vi "WriteStream ClientStreamTemplate.vi"(8 "error in":errorcluster, 10 "Request Data":cluster{"Numeric":dbl}, 11 "Call ID in":T1) -> (0 "error out":errorcluster, 2 "Success":bool, 3 "Call ID":T1)   [LabVIEW 2020, in "MeasurementLink Pin Map Client.lvlib"]
uses:
  <vilib>/gRPC/LabVIEW gRPC Library/Shared/grpcId.ctl
  bc3a45f8-3032-43b6-bbd2-58fc852009b1.vi
  9647bdd3-bda2-4565-bbb9-d670be58a455.vi
  <vilib>/gRPC/LabVIEW gRPC Library/Shared/TranslateGrpcError.vi
  <vilib>/gRPC/LabVIEW gRPC Library/Server API/Server/Get Server DLL Path.vi
  <vilib>/Utility/error.llb/Error Cluster From Error Code.vi
  <vilib>/Utility/error.llb/Simple Error Handler.vi
  MeasurementLink Pin Map Client.lvlib
  <vilib>/gRPC/LabVIEW gRPC Library/grpc-lvsupport-release.lvlib
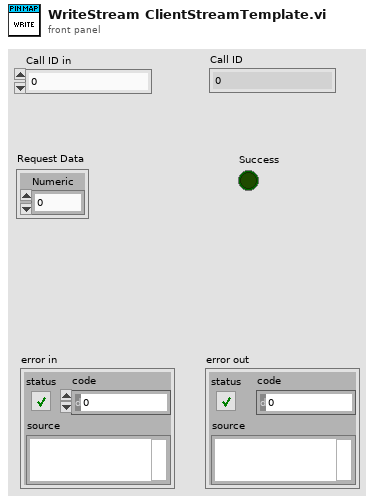
[diagram p1: front panel]
types:
  T1 = typedef "grpc-lvsupport-release.lvlib/grpcId.ctl" = u64
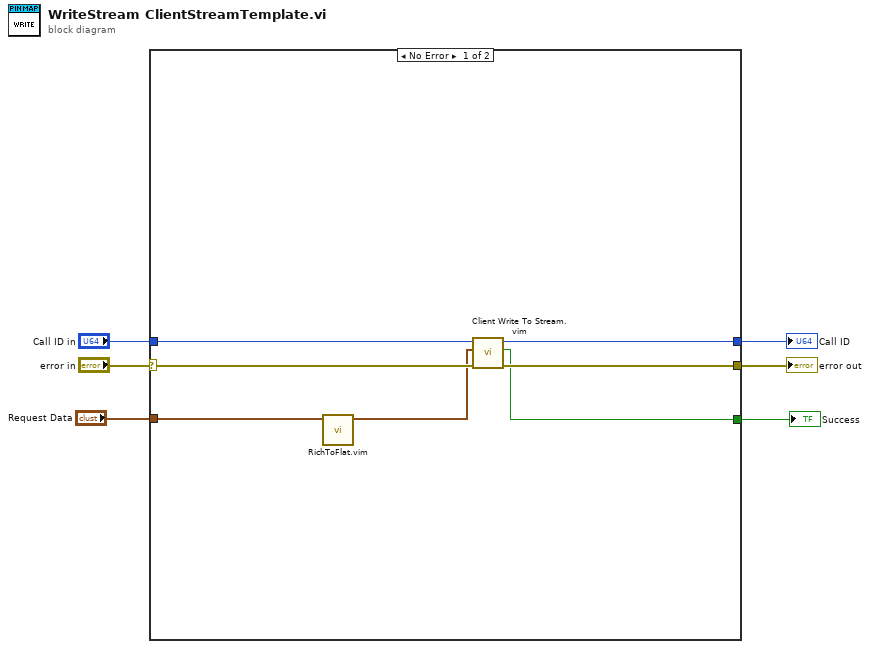
[diagram p0: block diagram]
diagram:
  n1 = case shown="No Error" "error in" {
    selector: "error in" -> [w13 w14]
    tunnel: [w12 w14] -> w5
    tunnel: "Call ID in" -> [w11 w15]
    tunnel: [w10 w15] -> w3
    tunnel: "Request Data" -> [w8 _]
    tunnel: [w9 _] -> w1
    frame No Error {
      n2 = call "RichToFlat.vim"("InputCluster"=w8) -> ("OutputCluster"=w7:cluster{"Numeric":dbl})  [unwired: 10 in]
      n3 = call "Client Write To Stream.vim"("error in"=w13, "Request Data"=w7, "Call ID in"=w11) -> ("error out"=w12:errorcluster, "Success"=w9:bool, "Call ID out"=w10:u64)  [unwired: 6 in]
    }
    frame Error {
    }
  }
  "error out" <- w5
  "Call ID" <- w3
  "Success" <- w1
